vi "Append Control Image to Report.vi"(0 "report in":refnum<class "NI_Word.lvclass">, 1 "alignment (default)":T2, 2 "image file type (.jpg)":enum16{".jpg", ".png"}(ring), 5 "image depth":T1=3 items=["B&W", "4 bits", "8 bits", "24 bits"], 7 "ctrl reference":refnum<vi>, 9 "description":string, 11 "error in (no error)":errorcluster, 12 "MS Office parameters":T3) -> (4 "report out":refnum<class "NI_Word.lvclass">, 8 "start out (Word)":i32, 10 "end out (Word)":i32, 15 "error out":errorcluster)   [LabVIEW 2023, in "NI_Word.lvclass"]
doc: "Creates an image of the front panel object specified in <B>Ctrl Reference</B> and appends it to a report."
uses:
  NI_Word.lvclass
  <vilib>/Utility/NIReport.llb/HTML Report Image Alignment.ctl
  <vilib>/Utility/NIReport.llb/NI_ReportGenerationCore.lvlib
  <vilib>/Utility/NIReport.llb/image depth.ctl
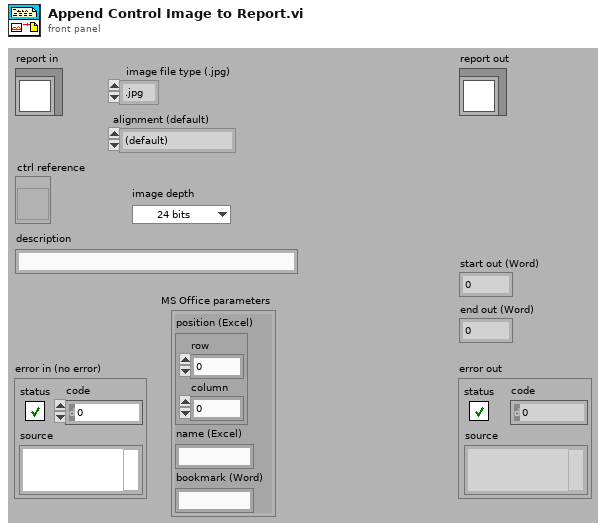
[diagram p1: front panel]
types:
  T1 = typedef "NI_ReportGenerationCore.lvlib/image depth.ctl" = u16
  T2 = typedef "NI_ReportGenerationCore.lvlib/HTML Report Image Alignment.ctl" = enum16{"(default)", "LEFT", "RIGHT", "TOP", "TEXTTOP", "MIDDLE", "ABSMIDDLE", "BASELINE", "BOTTOM", "ABSBOTTOM"}
  T3 = cluster{"position (Excel)":cluster{"row":i32, "column":i32}, "name (Excel)":string, "bookmark (Word)":string}
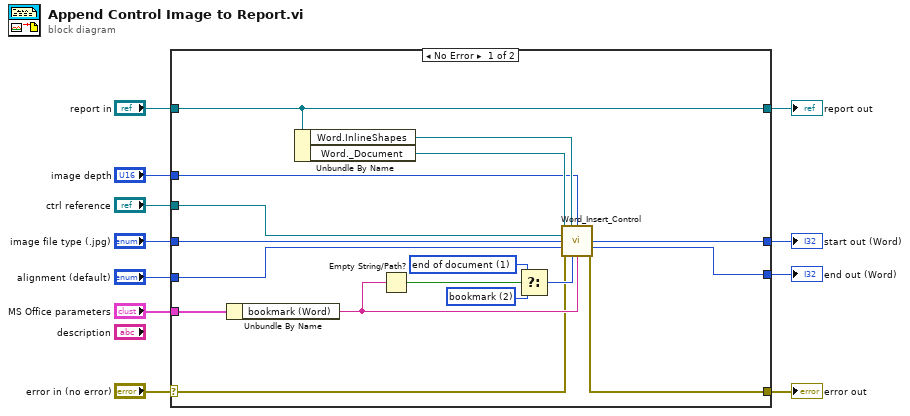
[diagram p0: block diagram]
diagram:
  n1 = case shown="No Error" "error in (no error)" {
    selector: "error in (no error)" -> [w19 w30]
    tunnel: [w18 w30] -> w10
    tunnel: [w21 w29] -> w8
    tunnel: "report in" -> [w21 w29]
    tunnel: "MS Office parameters" -> [w20 _]
    tunnel: "image file type (.jpg)" -> [w17 _]
    tunnel: "ctrl reference" -> [w16 _]
    tunnel: "alignment (default)" -> [w15 _]
    tunnel: [w14 _] -> w3
    tunnel: [w13 _] -> w2
    tunnel: "image depth" -> [w12 _]
    frame No Error {
      w22 = u16 2 items=["begining of document", "end of document", "bookmark", "custom"] ("Insertion point")
      w23 = u16 1 items=["begining of document", "end of document", "bookmark", "custom"] ("Insertion point")
      n2 = Unbundle By Name(w20) -> ("bookmark (Word)"=w28:string)
      n3 = Unbundle By Name(w21) -> ("Word.InlineShapes"=w25:refnum<k7>, "Word._Document"=w26:refnum<k7>)
      n4 = Empty String/Path?(string/path=w28) -> (empty?=w24:bool)
      n5 = Select(t=w23, s=w24, f=w22) -> (s? t:f=w27:u16)
      n6 = call <vilib>:"Word_Insert_Control.vi"("Word.Document"=w26, "Word.InlineShapes"=w25, "image depth"=w12, "Ctl Refnum"=w16, "image file type(.jpg)"=w17, "alignment (default)"=w15, "error in"=w19, "Insertion point"=w27, "bookmark name"=w28) -> ("Start out"=w14:i32, "End out"=w13:i32, "error out"=w18:errorcluster)  [unwired: 4 out]
    }
    frame Error {
    }
  }
  "error out" <- w10
  "report out" <- w8
  "start out (Word)" <- w3
  "end out (Word)" <- w2
